vi "Set Component Settings By ID.vi"(8 "error in (no error)":errorcluster, 9 "component settings":T2[](array[typedef]), 10 "settings id":T1={"plugin"=-1, "thread"=-1, "group"=-1, "transfer"=-1, "channel"=-1}, 11 "Runtime Configuration in":refnum<class "Core Configuration.lvclass">) -> (0 "error out":errorcluster, 3 "Runtime Configuration out":refnum<class "Core Configuration.lvclass">)   [LabVIEW 2021, in "DSF Core.lvlib" / "Core Configuration.lvclass"]
uses:
  Core Configuration.lvclass
  Typedefs/DSF Settings Info.ctl
  Typedefs/DSF Configuration ID.ctl
  DSF Core.lvlib
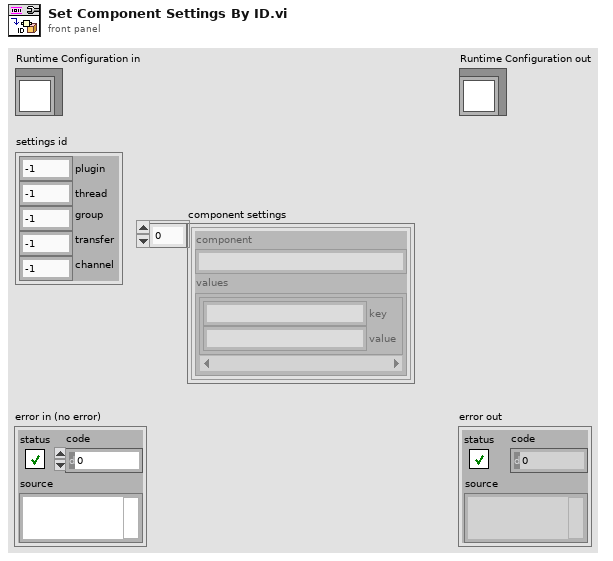
[diagram p1: front panel]
types:
  T1 = typedef "DSF Core.lvlib/DSF Configuration ID.ctl" = cluster{"plugin":i32, "thread":i32, "group":i32, "transfer":i32, "channel":i32}
  T2 = typedef "DSF Core.lvlib/DSF Settings Info.ctl" = cluster{"component":string, "values":cluster{"key":string, "value":string}[]}
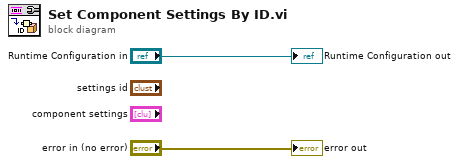
[diagram p0: block diagram]
diagram:
  "error out" <- "error in (no error)"
  "Runtime Configuration out" <- "Runtime Configuration in"
